vi "Init_DAQ.vi"(8 "error in":errorcluster caption="entrée d'erreur") -> (0 "error out":errorcluster caption="sortie d'erreur")   [LabVIEW 2026]
uses:
  Controls/TypeDef_FGV.ctl
  <vilib>/DAQmx/create/channels.llb/DAQmx Create Channel (CO-Pulse Generation-Time).vi
  FGV/FGV_DAQ_CO_Task.vi
  <vilib>/DAQmx/create/channels.llb/DAQmx Create Channel (DI-Digital Input).vi
  <vilib>/DAQmx/configure/timing.llb/DAQmx Timing (Change Detection).vi
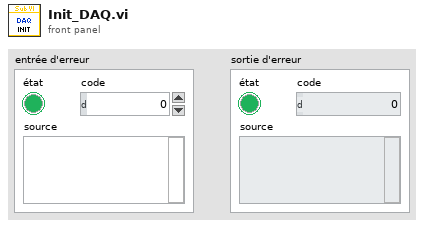
[diagram p1: front panel]
types:
  T1 = typedef "TypeDef_FGV.ctl" = enum16{"Initialize", "Write", "Read"}
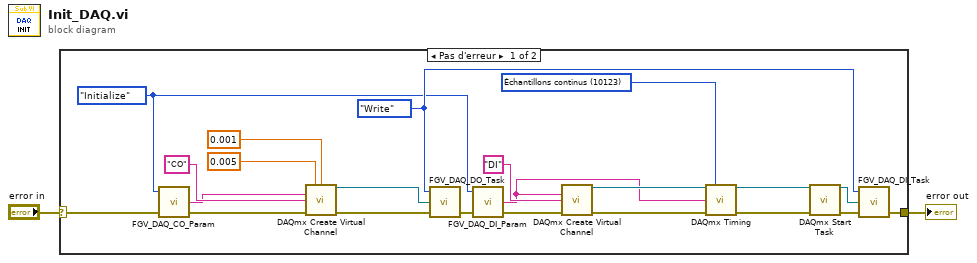
[diagram p0: block diagram]
diagram:
  n1 = case shown="Pas d'erreur" "error in" {
    selector: "error in" -> [w5 w25]
    tunnel: [w18 w25] -> w1
    frame No Error {
      w14 = 10123 items=["Échantillons finis"=10178, "Échantillons continus"=10123, "Point par point avec cadencement matériel"=12522] ("sample mode")
      w6 = TypeDef_FGV."Initialize" ("Action")
      w19 = TypeDef_FGV."Write" ("Action")
      n2 = call "FGV_DAQ_CO_Param.vi"("error in"=w5, "Action"=w6) -> ("error out"=w4:errorcluster, "CO line"=w3:tag)  [unwired: 2 in]
      n3 = call-poly <vilib>:"DAQmx Create Virtual Channel.vi"("high time"=0.005, "low time"=0.001, "counter"=w3, "name to assign"="CO", "error in"=w4) -> ("task out"=w22:refnum<k21>, "error out"=w23:errorcluster)  [unwired: 9 in]
      n4 = call "FGV_DAQ_DO_Task.vi"("error in"=w23, "CO task"=w22, "Action"=w19) -> ("error out"=w21:errorcluster)  [unwired: 1 in, 1 out]
      n5 = call "FGV_DAQ_DI_Param.vi"("error in"=w21, "Action"=w6) -> ("error out"=w20:errorcluster, "DI line"=w9:tag)  [unwired: 2 in]
      n6 = call-poly <vilib>:"DAQmx Create Virtual Channel.vi"("lines"=w9, "name to assign"="DI", "error in"=w20) -> ("task out"=w16:refnum<k21>, "error out"=w15:errorcluster)  [unwired: 11 in]
      n7 = call-poly <vilib>:"DAQmx Timing.vi"("task/channels in"=w16, "sample mode"=w14, "rising edge physical channels"=w9, "error in"=w15) -> ("task out"=w13:refnum<k21>, "error out"=w12:errorcluster)  [unwired: 10 in]
      n8 = call <vilib>:"DAQmx Start Task.vi"("task/channels in"=w13, "error in"=w12) -> ("task out"=w11:refnum<k21>, "error out"=w10:errorcluster)  [unwired: 12 in]
      n9 = call "FGV_DAQ_DI_Task.vi"("error in"=w10, "DI task"=w11, "Action"=w19) -> ("error out"=w18:errorcluster)  [unwired: 1 in, 1 out]
    }
    frame Error {
    }
  }
  "error out" <- w1
